vi "Ist mit Soll vergleichen Alarme.vi"(8 "error in (no error)":errorcluster caption="Fehler (Eingang, kein Fehler)", 11 "mini8 Steuerung PNS Eingang":refnum<class "mini8 Steuerung PNS.lvclass">) -> (0 "error out":errorcluster caption="Fehler (Ausgang)", 2 "Werte":cluster{u16[], u16[]}, 3 "mini8 Steuerung PNS Ausgang":refnum<class "mini8 Steuerung PNS.lvclass">)   [LabVIEW 2020, in "mini8 Steuerung PNS.lvclass"]
uses:
  mini8 Steuerung PNS.lvclass
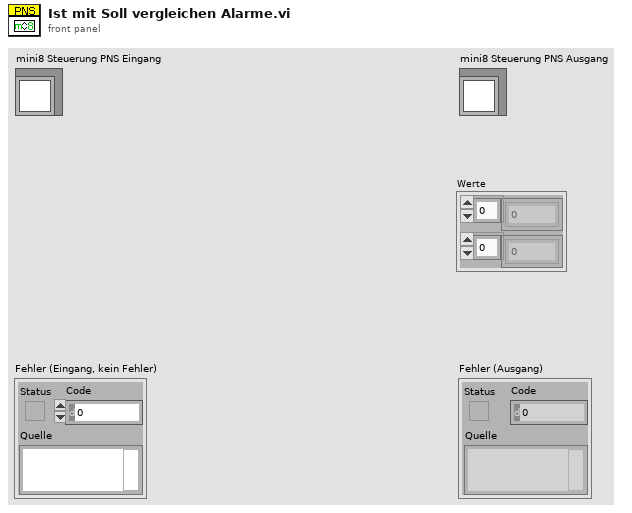
[diagram p1: front panel]
types:
  T1 = typedef "Steuerung PNS.lvclass/Anlegengrenzwerte PNS.ctl" = cluster{"Filter:":T2, "Ventilplatte:":T2, "Heizleitung 1:":T2, "Heizleitung 2:":T2, "Heizleitung 3:":T2, "Heizleitung 4:":T2, "Heizleitung 5:":T2, "Heizleitung 6:":T2}
  T2 = typedef "Steuerung PNS.lvclass/Anlagengrenzwerte Parameteranzeige.ctl" = cluster{"Sollwert":T3, "Warn-Min":T3, "Warn-Max":T3, "Abschalt-Min":T3, "Abschalt-Max":T3, "Regler":u16, "AnlagenParameter":string}
  T3 = typedef "Zahlen-Eingabefeld.ctl" = sgl
  T4 = typedef "Steuerung PNS.lvclass/Alarme.ctl" = cluster{"Alarm Filter max":u16, "Alarm Filter min":u16, "Alarm Ventilplatte max":u16, "Alarm Ventilplatte min":u16, "Alarm HL1 max":u16, "Alarm HL1 min":u16, "Alarm HL2 max":u16, "Alarm HL2 min":u16, "Alarm HL3 max":u16, "Alarm HL3 min":u16, "Alarm HL4 max":u16, "Alarm HL4 min":u16, "Alarm HL5 max":u16, "Alarm HL5 min":u16, "Alarm HL6 max":u16, "Alarm HL6 min":u16}
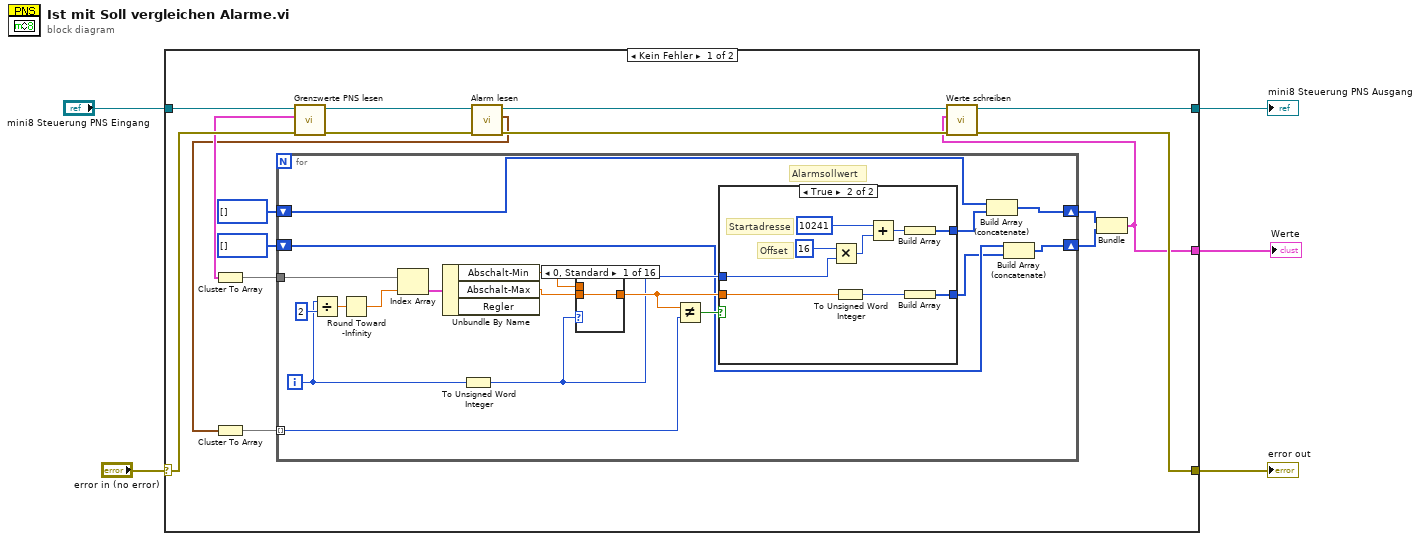
[diagram p0: block diagram]
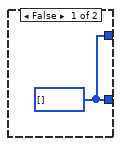
[diagram p2: hidden frame]
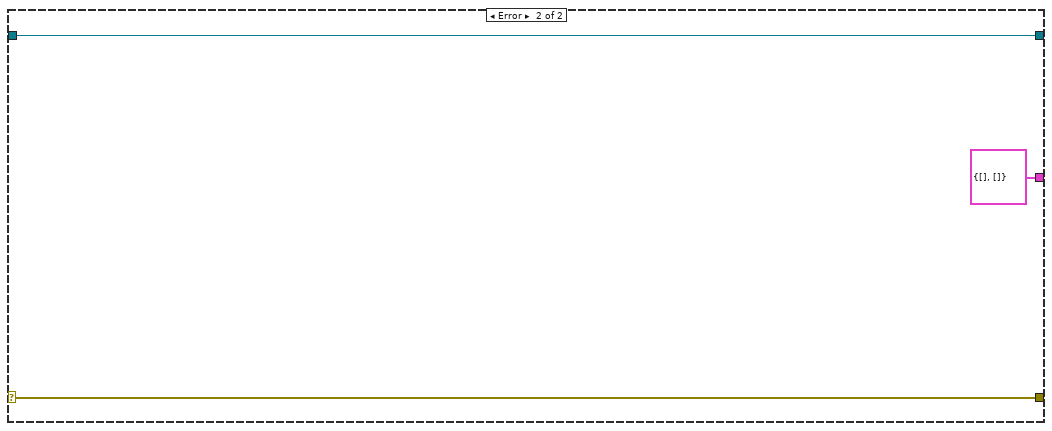
[diagram p18: hidden frame]
diagram:
  n1 = case shown="Kein Fehler" "error in (no error)" {
    selector: "error in (no error)" -> [w16 w69]
    tunnel: [w15 w69] -> w4
    tunnel: [w18 w68] -> w2
    tunnel: "mini8 Steuerung PNS Eingang" -> [w22 w68]
    tunnel: [w8 cluster{u16[], u16[]} {[], []}] -> w1
    frame No Error {
      n2 = call-dynamic "Grenzwerte PNS lesen.vi"("error in (no error)"=w16, "Steuerung PNS (Eingang)"=w22) -> ("error out"=w19:errorcluster, "Grenzwerte PNS"=w14:T1, "Steuerung PNS (Ausgang)"=w21:refnum<class "mini8 Steuerung PNS.lvclass">)  [unwired: 7 in]
      n3 = Cluster To Array(cluster=w14) -> (array=w13:T2[])
      n4 = call-dynamic "Alarm lesen.vi"("error in (no error)"=w19, "Steuerung PNS (Eingang)"=w21) -> ("error out"=w17:errorcluster, "Alarm"=w12:T4, "Steuerung PNS (Ausgang)"=w20:refnum<class "mini8 Steuerung PNS.lvclass">)  [unwired: 7 in]
      n5 = Cluster To Array(cluster=w12) -> (array=w11:u16[])
      n6 = for {
        tunnel: w13 -> [w40]
        shift-right: [w27] -> w10
        shift-left: u16[] [] -> [w29]
        shift-right: [w26] -> w9
        shift-left: u16[] [] -> [w25]
        tunnel: w11 -> [w23] mode=indexing
        i -> [w31]
        # "Alarmsollwert"
        n7 = Divide(x=w31, y=2) -> (x/y=w37:dbl)
        n8 = Round Toward -Infinity(1:w37) -> (0:w36:dbl)
        n9 = Index Array(array=w40, index=w36) -> (element=w39:T2)
        n10 = Unbundle By Name(w39) -> ("Abschalt-Min"=w35:T3, "Abschalt-Max"=w34:T3)  [unwired: 1 out]
        n11 = To Unsigned Word Integer(number=w31) -> (unsigned 16bit integer=w30:u16)
        n12 = case shown="0, Standard" w30 {
          tunnel: w35 -> [_ w52 _ w54 _ w56 _ w58 _ w60 _ w62 _ w64 _ w66]
          tunnel: w34 -> [w51 _ w53 _ w55 _ w57 _ w59 _ w61 _ w63 _ w65 _]
          tunnel: [w51 w52 w53 w54 w55 w56 w57 w58 w59 w60 w61 w62 w63 w64 w65 w66] -> w33
          frame 0, Default {
          }
          frame 1 {
          }
          frame 2 {
          }
          frame 3 {
          }
          frame 4 {
          }
          frame 5 {
          }
          frame 6 {
          }
          frame 7 {
          }
          frame 8 {
          }
          frame 9 {
          }
          frame 10 {
          }
          frame 11 {
          }
          frame 12 {
          }
          frame 13 {
          }
          frame 14 {
          }
          frame 15 {
          }
        }
        n13 = Not Equal?(x=w33, y=w23) -> (x != y?=w32:bool)
        n14 = case shown="True" w32 {
          tunnel: w33 -> [_ w46]
          tunnel: [w41 w44] -> w28
          tunnel: [w41 w43] -> w24
          tunnel: w30 -> [_ w42]
          frame False {
            w41 = u16[] []
          }
          frame True {
            # "Offset"
            # "Startadresse"
            n15 = Multiply(x=u16 16, y=w42) -> (x*y=w50:u16)
            n16 = To Unsigned Word Integer(number=w46) -> (unsigned 16bit integer=w45:u16)
            n17 = Add(x=u16 10241, y=w50) -> (x+y=w47:u16)
            n18 = Build Array(w47) -> (w44:u16[])
            n19 = Build Array(w45) -> (w43:u16[])
          }
        }
        n20 = Build Array (concatenate)(w29, w28) -> (w27:u16[])
        n21 = Build Array (concatenate)(w25, w24) -> (w26:u16[])
      }
      n22 = Bundle(w10, w9) -> (w8:cluster{u16[], u16[]})  [unwired: 1 in]
      n23 = call-dynamic "Werte schreiben.vi"("error in (no error)"=w17, "Werte"=w8, "Steuerung PNS (Eingang)"=w20) -> ("error out"=w15:errorcluster, "Steuerung PNS (Ausgang)"=w18:refnum<class "mini8 Steuerung PNS.lvclass">)  [unwired: 7 in]
    }
    frame Error {
    }
  }
  "error out" <- w4
  "mini8 Steuerung PNS Ausgang" <- w2
  "Werte" <- w1
